vi "MB_PLC Comm Tester.vi"() -> ()   [LabVIEW 2018]
uses:
  Types/MB Ref Range_Cluster.ctl
  MB PLC Client.lvclass
  Data/MB Data Block.lvclass
  Types/MB Data Types_Enum.ctl
  Types/TCP Config_Cluster.ctl
  Types/PLC Config_Cluster.ctl
  Types/Serial Config_Cluster.ctl
  MB PLC Client.lvclass/MB PLC Client.ctl
  <vilib>/Plasmionique/MB Master/MB_ADU/MB_ADU.lvclass/MB_ADU.ctl
  Read MB session.vi
  <vilib>/Plasmionique/MB Master/MB_ADU/Read TX Data.vi
  <vilib>/Plasmionique/MB Master/MB_ADU/Read RX Data.vi
  <vilib>/Plasmionique/MB Master/MB_ADU/Read TX Timestamp.vi
  Read Poll List.vi
  c75dd57c-5bee-49d0-a77c-1ce558688484.vi
  28e4650d-529a-4e98-aa34-076f74409b59.vi
  46e13ee2-e094-4c5a-84fa-59b6ca3f2090.vi
  7f289292-5569-4f0d-9d85-fdf3f2f5d33f.vi
  734f5e53-c859-40ca-a5fa-c5cf108e6d6f.vi
  c81834c4-dabb-43f2-ab20-ca57d7a4baed.vi
  a754e2c8-79f3-43f7-b060-ecd024e2671e.vi
  Read PLC Config.vi
  0477ca1b-c906-4639-9e15-2d9a6e8c9738.vi
  7c55f3c8-79e0-44ec-bef0-26051c578f47.vi
  79f87e31-4c7f-45de-9eca-f5432d7d6e87.vi
  cd595503-730d-404a-9a2b-57208e76ed7d.vi
  b1a69734-ed15-4636-bb1c-7f177049bbcd.vi
  caadcf0a-5e3c-445f-9426-b9186ab7a80d.vi
  8821aff1-d05f-48ce-8825-efee275c2a12.vi
  Write Poll List.vi
  28e4650d-529a-4e98-aa34-076f74409b59.vi/fa59bfe1-0120-4885-ac93-9d9ea70f91fc.vi
  46e13ee2-e094-4c5a-84fa-59b6ca3f2090.vi/4d1e8f78-cfda-4438-959d-f24f6f91643b.vi
  7f289292-5569-4f0d-9d85-fdf3f2f5d33f.vi/b046c757-7f56-4393-a6ce-7771a5783ef5.vi
  734f5e53-c859-40ca-a5fa-c5cf108e6d6f.vi/f0ac0d71-d2d5-4ce4-9473-de91a0dd1fbe.vi
  c81834c4-dabb-43f2-ab20-ca57d7a4baed.vi/f658b24b-f49e-4e74-aef7-a7a595d7420c.vi
  a754e2c8-79f3-43f7-b060-ecd024e2671e.vi/da5e4fd7-561c-4cb8-8319-9a995167b5c8.vi
  0477ca1b-c906-4639-9e15-2d9a6e8c9738.vi/f491cc9f-02c6-4ff0-92db-d4c2192e9176.vi
  Read Data Block.vi
  7c55f3c8-79e0-44ec-bef0-26051c578f47.vi/6d4b17d2-94aa-44ea-9a19-d0a6b7bc1155.vi
  79f87e31-4c7f-45de-9eca-f5432d7d6e87.vi/0bbcd01c-01b7-4bc8-b012-ee89d531728c.vi
  cd595503-730d-404a-9a2b-57208e76ed7d.vi/d20b6ab7-2084-4e8d-b3bf-d366641d9b9f.vi
  b1a69734-ed15-4636-bb1c-7f177049bbcd.vi/f504e7b8-0e68-4180-b08b-6a52a05c8892.vi
  caadcf0a-5e3c-445f-9426-b9186ab7a80d.vi/238819c2-a843-4790-bae3-c60b5cb0f74c.vi
  8821aff1-d05f-48ce-8825-efee275c2a12.vi/d735e59b-17a8-402d-8d0a-4356da9fddb7.vi
  28e4650d-529a-4e98-aa34-076f74409b59.vi/fa59bfe1-0120-4885-ac93-9d9ea70f91fc.vi/6bf269be-e776-4970-9958-56c4dbea2623.vi
  46e13ee2-e094-4c5a-84fa-59b6ca3f2090.vi/4d1e8f78-cfda-4438-959d-f24f6f91643b.vi/79965a6c-bbeb-417c-a67a-cf8599a87570.vi
  7f289292-5569-4f0d-9d85-fdf3f2f5d33f.vi/b046c757-7f56-4393-a6ce-7771a5783ef5.vi/c7e8f3d7-7cb7-4e11-b1a0-06c415cc4c12.vi
  734f5e53-c859-40ca-a5fa-c5cf108e6d6f.vi/f0ac0d71-d2d5-4ce4-9473-de91a0dd1fbe.vi/b105db0b-c665-47de-b7cd-89c5a82b0a3a.vi
  c81834c4-dabb-43f2-ab20-ca57d7a4baed.vi/f658b24b-f49e-4e74-aef7-a7a595d7420c.vi/682b31c2-d550-4a42-88b0-f85749b69dfb.vi
  a754e2c8-79f3-43f7-b060-ecd024e2671e.vi/da5e4fd7-561c-4cb8-8319-9a995167b5c8.vi/d8f5afb1-d2bc-4e28-9ddd-dab29005bbc2.vi
  7c55f3c8-79e0-44ec-bef0-26051c578f47.vi/6d4b17d2-94aa-44ea-9a19-d0a6b7bc1155.vi/88869970-30da-475b-b9b2-9c3da2a1dedf.vi
  79f87e31-4c7f-45de-9eca-f5432d7d6e87.vi/0bbcd01c-01b7-4bc8-b012-ee89d531728c.vi/679bbca3-05f9-4675-a6af-c2baf730c5e7.vi
  cd595503-730d-404a-9a2b-57208e76ed7d.vi/d20b6ab7-2084-4e8d-b3bf-d366641d9b9f.vi/8995d4bf-6152-44d7-9e95-9528b4a066ce.vi
  b1a69734-ed15-4636-bb1c-7f177049bbcd.vi/f504e7b8-0e68-4180-b08b-6a52a05c8892.vi/fec356c3-a4ba-4058-8d4b-0e5c98c3ed52.vi
  caadcf0a-5e3c-445f-9426-b9186ab7a80d.vi/238819c2-a843-4790-bae3-c60b5cb0f74c.vi/1018f8a3-db30-48a7-bdd6-e7d4ad86f488.vi
  8821aff1-d05f-48ce-8825-efee275c2a12.vi/d735e59b-17a8-402d-8d0a-4356da9fddb7.vi/efbd7a58-b214-41d9-909a-8167e3be0071.vi
  <vilib>/Utility/error.llb/Error Cluster From Error Code.vi
  Write Coils_Cached.vi
  Write Holding Registers_Cached.vi
  <vilib>/Plasmionique/MB Master/MB_Master/MB_Master.lvclass
  <vilib>/Plasmionique/MB Master/MB_ADU/MB_ADU.lvclass
  MB PLC Client.lvlib
panel:
  out "Poll Count":u32
  out "Last Error Time":string
  in  "Tab Control 2":T1(tab)
  in  "Swap Words":bool
  in  "Reference Format":u16(ring)=5 items=["4 Digits"=4, "5 Digits"=5, "6 Digits"=6]
  in  "Open":bool
  in  "Close":bool
  in  "Type":enum16{"Serial", "TCP"}(ring) caption="Connection Type"
  in  "Tab Control":enum32{"Page 1", "Page 2"}(tab)
  in  "Retries":u8=1
  in  "Timeout (ms)":u32=300
  in  "Flow Control":u16(ring) items=["None", "XON/XOFF", "RTS/CTS", "XON/XOFF & RTS/CTS", "DTR/DSR", "XON/XOFF & DTR/DSR"]
  in  "Parity":u16(ring) items=["None", "Odd", "Even", "Mark", "Space"]
  in  "Stop Bits":u16(ring)=10 items=["1.0"=10, "1.5"=15, "2.0"=20]
  in  "Baud Rate (bps)":u32(ring)=19200 items=["9600"=9600, "19200"=19200, "38400"=38400, "57600"=57600, "115200"=115200, "460800"=460800, "921600"=921600]
  in  "Slave Address":u8=1
  in  "Mode":enum16{"RTU", "ASCII"}(ring)
  in  "COM Port":refnum<visa-resource-name>
  in  "TCP_Port":u16=502 caption="Port"
  in  "IP Address":string="localhost"
  in  "TCP_Timeout":i32=10000 caption="Timeout (ms)"
  in  "TCP_Slave ID":u8=255 caption="Slave ID" format="%.0x"
  in  "Poll Period (ms)":i32=1000
  in  "MaxPollGap":i32=1
  out "Message Log":T2(array[cluster]) {"dt" format="%d ms"; "Time" format="%<%H:%M:%S%1u>T"}
  out "Last Error Status":errorcluster
  out "Poll List":T3[](array[typedef])
  in  "New Value":dbl
  in  "Remove All":bool
  out "Register Type":string
  in  "Name":string
  in  "Data Type":T4(ring)
  in  "Starting Reference":u32 format="%05d"
  in  "Write Value":bool
  in  "Remove":bool
  in  "Add":bool
  in  "Watchlist":i32(listbox)
  out "Input Registers":u16[](array[numeric])
  out "Holding Registers":u16[](array[numeric]) format="%.0x"
  out "Discrete Inputs":bool[](array[boolean])
  out "Coils":bool[](array[boolean])
  out "Open?":bool caption="Connected"
  # "Communication Settngs"
  # "Communication Status"
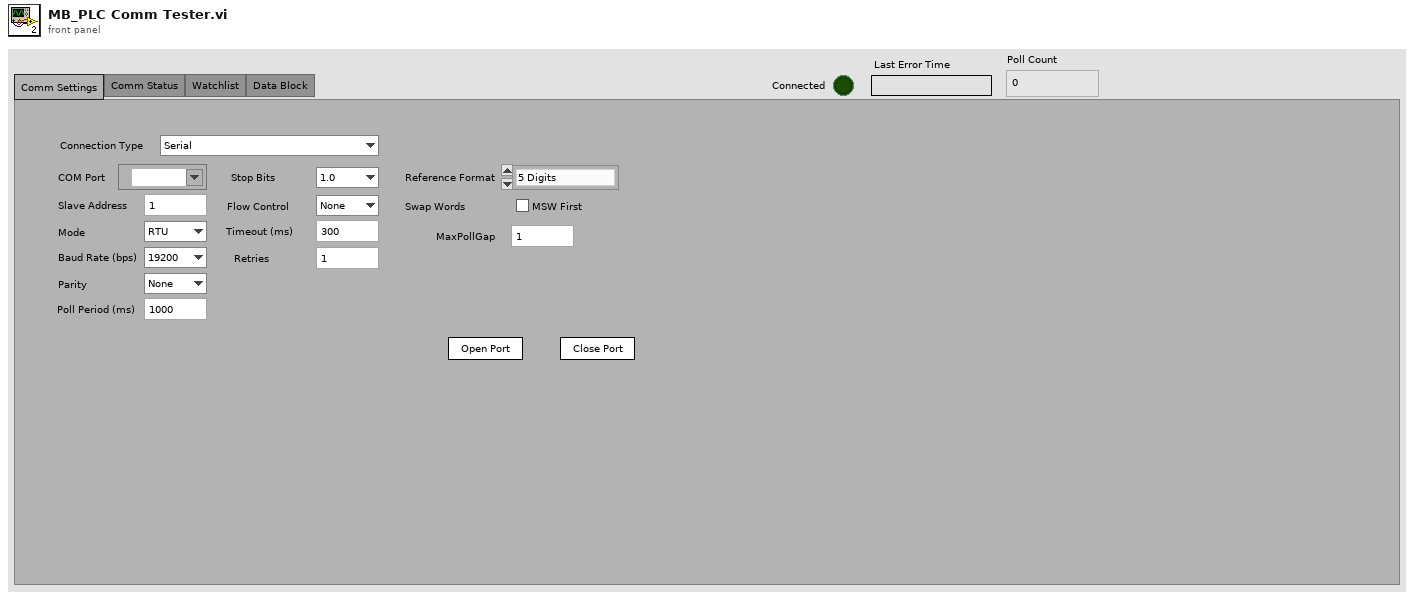
[diagram p1: front panel]
types:
  T1 = enum32{"Comm Settings", "Comm Status", "Watchlist", "Data Block"}
  T2 = cluster{"Time":timestamp, "TX":string, "RX":string, "dt":dbl}[]
  T3 = typedef "MB PLC Client.lvlib/MB Ref Range_Cluster.ctl" = cluster{"Start":u32, "Qty":u16}
  T4 = enum16{"Bool", "U16", "U32", "I16", "I32", "SGL", "DBL"}
  T5 = cluster{"Timestamp":timestamp, "TX":string, "RX":string, "dt":u32}
  T6 = typedef "MB PLC Client.lvlib/MB Data Types_Enum.ctl" = enum16{"Bool", "U16", "U32", "I16", "I32", "SGL", "DBL"}
  T7 = cluster{"Open":bool, "BinData":bool, "WatchList":cluster{"Name":string, "Reference":u32, "Data Type":T6, "Value":dbl}[], "Poll Count":u32}
  T8 = typedef "MB PLC Client.lvlib/Serial Config_Cluster.ctl" = cluster{"COM Port":string, "Slave ID":u8, "baud rate (bps)":u32, "Mode":enum16{"RTU", "ASCII"}, "Parity":u16, "Flow Control":u16, "Timeout":u32, "Retries":u8, "Stop Bits":u16}
  T9 = typedef "MB PLC Client.lvlib/PLC Config_Cluster.ctl" = cluster{"Use TCP":bool, "Reference Format":u16, "Swap Words":bool, "Poll List":T3[]}
  T10 = typedef "MB PLC Client.lvlib/TCP Config_Cluster.ctl" = cluster{"IP Address":string, "Port":u16, "Slave ID":i8, "Timeout":i32}
  T11 = cluster{"Name":string, "Reference":u32, "Data Type":T6, "Value":dbl}
  T12 = cluster{"Properties:TX Timestamp":timestamp, "string":string, "string":string, u32}
  T13 = cluster{"Name":string, "Reference":u32, "Data Type":T6, "Value":dbl}[]
  T14 = typedef "MB PLC Client.lvlib/Reference Types_Enum.ctl" = enum16{"Coil", "Discrete Input", "Input Register", "Holding Register", "Invalid"}
  T15 = cluster{"Timestamp":timestamp, "TX":string, "RX":string, "dt":u32}[]
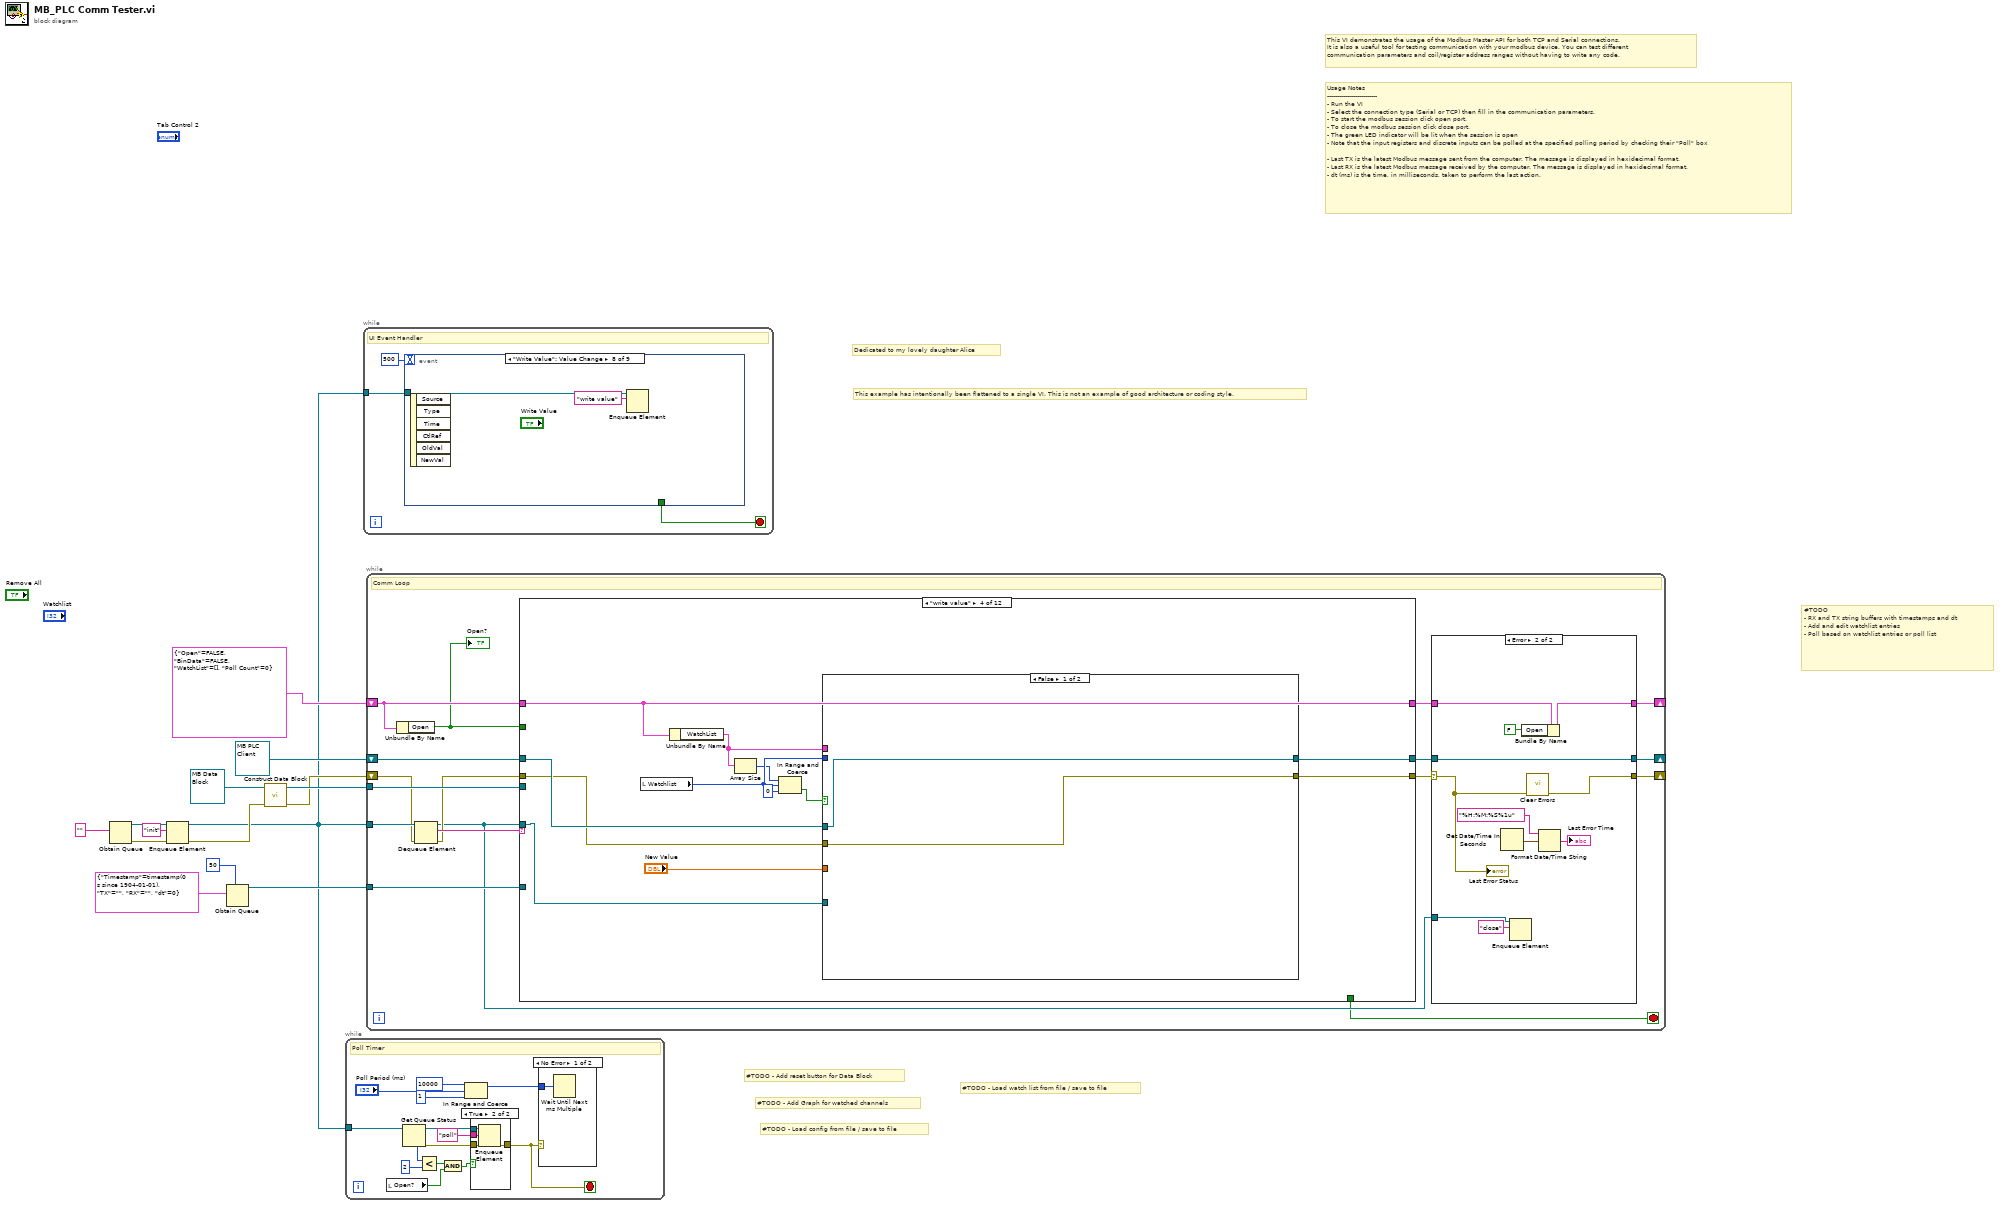
[diagram p0: block diagram]
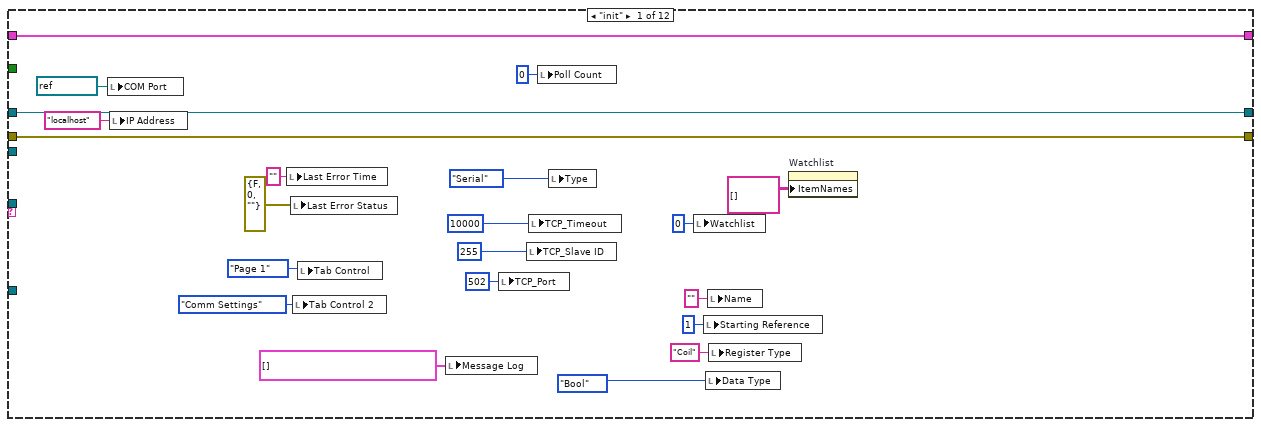
[diagram p5: hidden frame]
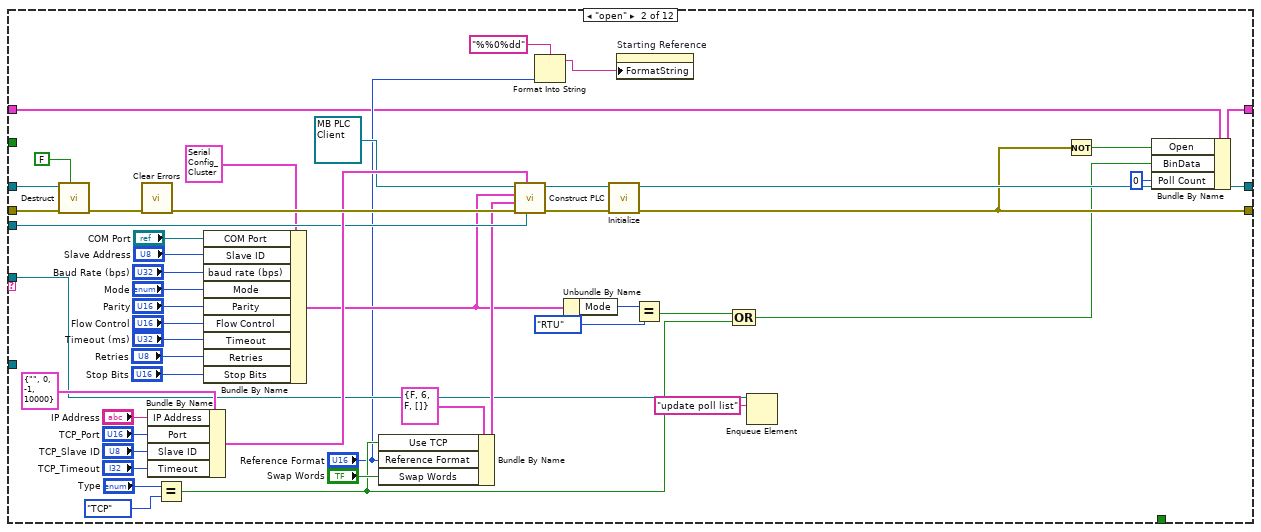
[diagram p6: hidden frame]
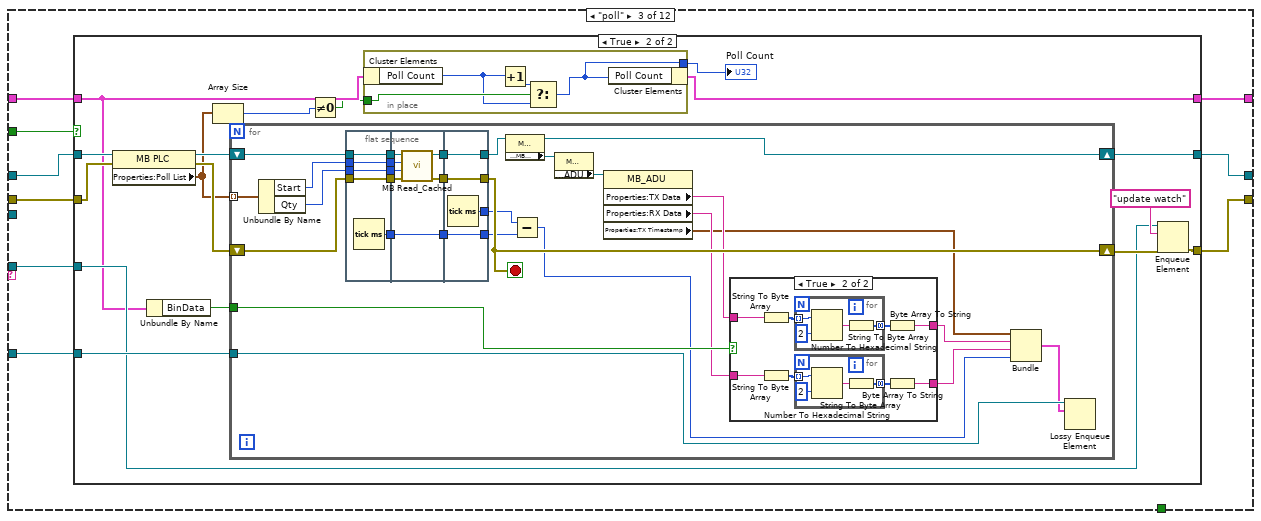
[diagram p7: hidden frame]
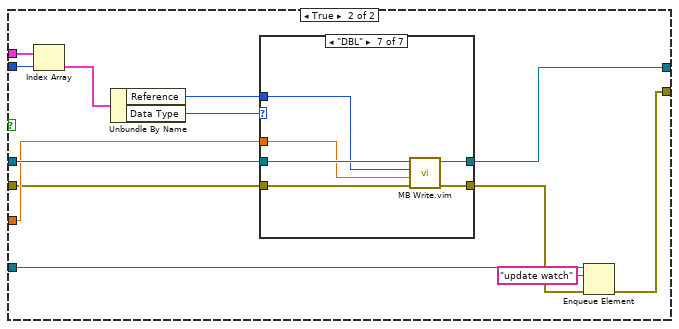
[diagram p10: hidden frame]
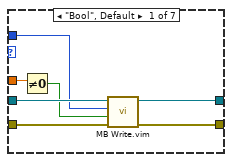
[diagram p11: hidden frame]
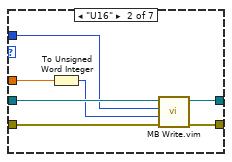
[diagram p12: hidden frame]
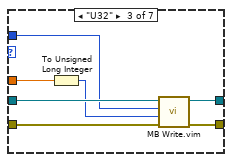
[diagram p13: hidden frame]
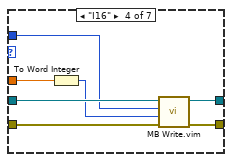
[diagram p14: hidden frame]
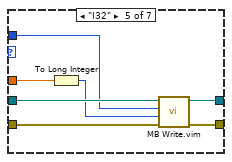
[diagram p15: hidden frame]
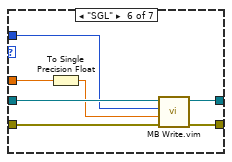
[diagram p16: hidden frame]
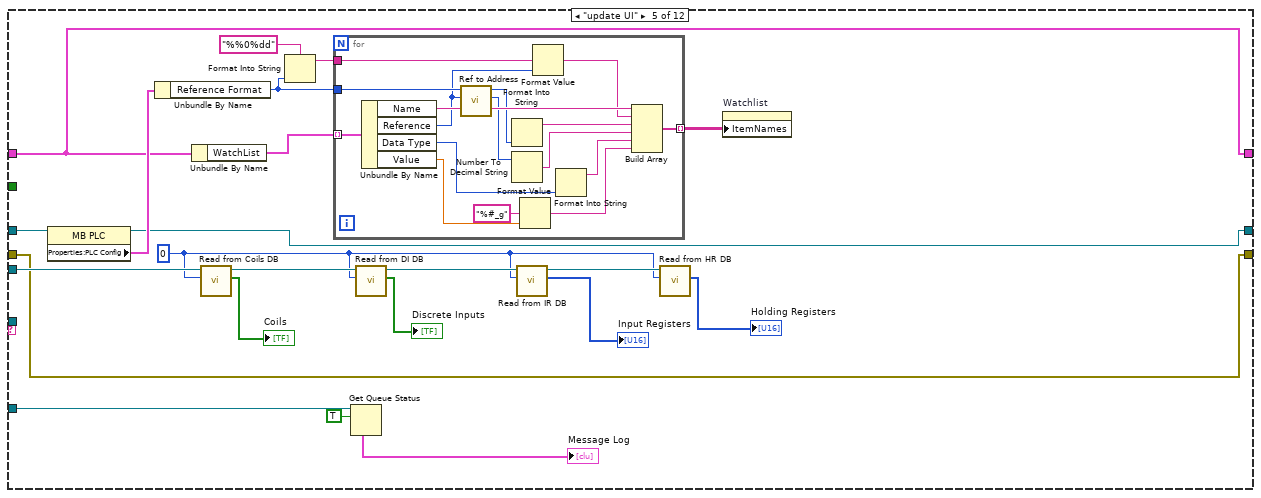
[diagram p17: hidden frame]
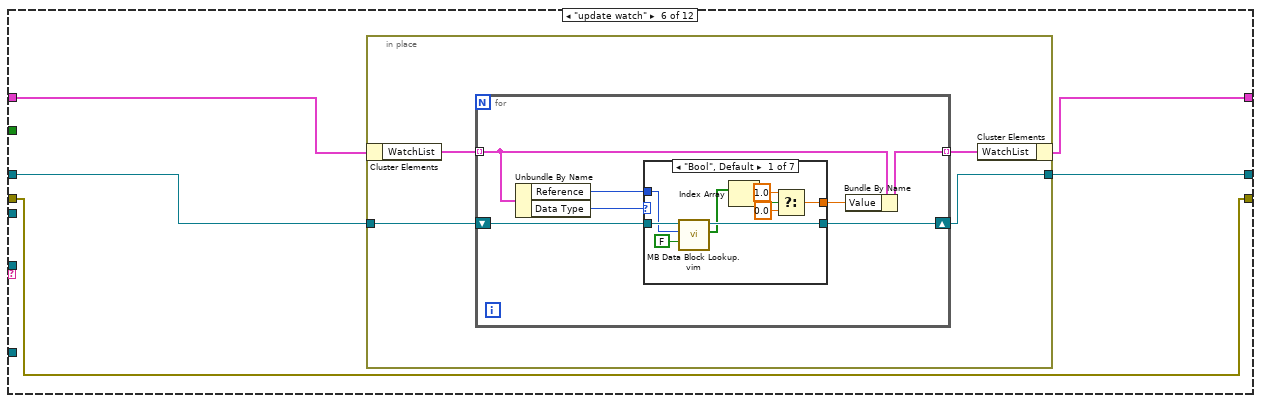
[diagram p18: hidden frame]
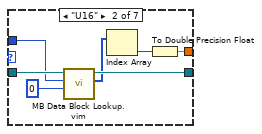
[diagram p19: hidden frame]
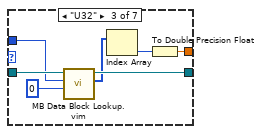
[diagram p20: hidden frame]
diagram:
  # "#TODO - Load watch list from file / save to file"
  # "#TODO - Load config from file / save to file"
  # "#TODO - Add Graph for watched channels"
  # "#TODO - Add reset button for Data Block"
  # "This example has intentionally been flattened to a single VI. This is not an example of good architecture or coding style."
  # "Dedicated to my lovely daughter Alice"
  # "#TODO\n- RX and TX string buffers with timestamps and dt\n- Add and edit watchlist entries\n- Poll based on watchlist entries or poll list"
  # "Usage Notes\n-------------------------\n- Run the VI\n- Select the connection type (Serial or TCP) then fill in the communication parameters.\n- To start the modbus session click open port.\n- To close the modbus session click close port.\n- The green LED indicator will be lit when the session is open\n- Note that the input registers and discrete inputs can be polled at the specified polling period by checking their \"Poll\" box\n\n- Last TX is the latest Modbus message sent from the computer. The message is displayed in hexidecimal format.\n- Last RX is the latest Modbus message received by the computer. The message is displayed in hexidecimal format. \n- dt (ms) is the time, in milliseconds, taken to perform the last action."
  # "This VI demonstrates the usage of the Modbus Master API for both TCP and Serial connections.\nIt is also a useful tool for testing communication with your modbus device. You can test different\ncommunication parameters and coil/register address ranges without having to write any code."
  n1 = Obtain Queue(element data type="") -> (queue out=w8:refnum<queue>, error out=w10:errorcluster)  [unwired: 4 in, 1 out]
  n2 = Enqueue Element(queue=w8, element="init", error in (no error)=w10) -> (queue out=w1:refnum<queue>, error out=w6:errorcluster)  [unwired: 1 in, 1 out]
  n3 = Obtain Queue(max queue size (-1, unlimited)=50, element data type=T5 {"Timestamp"=timestamp(0 s since 1904-01-01), "TX"="", "RX"="", "dt"=0}) -> (queue out=w2:refnum<queue>)  [unwired: 3 in, 2 out]
  n4 = call-dynamic "Construct Data Block.vi"("error in (no error)"=w6, "Modbus Data Store in"=refnum<class "MB Data Block.lvclass"> refnum ("MB Data Block (default)")) -> ("error out"=w5:errorcluster, "Modbus Data Store out"=w12:refnum<class "MB Data Block.lvclass">)  [unwired: 8 in]
  n5 = while {
    tunnel: w1 -> [w28]
    stop <- w19 stop-if-true
    # "Poll Timer"
    n6 = local read "Open?"() -> (w16:bool)
    n7 = Get Queue Status(queue=w28) -> (queue out=w20:refnum<queue>, error out=w21:errorcluster, # elements in queue=w27:i32)  [unwired: 2 in, 5 out]
    n8 = Less?(x=w27, y=2) -> (x < y?=w17:bool)
    n9 = And(x=w17, y=w16) -> (x .and. y?=w15:bool)
    n10 = In Range and Coerce(upper limit=10000, x="Poll Period (ms)", lower limit=1) -> (coerced(x)=w22:i32)  [unwired: 1 out]
    n11 = case shown="True" w15 {
      tunnel: w21 -> [w29 w33]
      tunnel: w20 -> [_ w32]
      tunnel: [w29 w31] -> w19
      tunnel: "poll" -> [_ w30]
      frame False {
      }
      frame True {
        n12 = Enqueue Element(queue=w32, element=w30, error in (no error)=w33) -> (error out=w31:errorcluster)  [unwired: 1 in, 2 out]
      }
    }
    n13 = case shown="No Error" w19 {
      tunnel: w22 -> [w34 _]
      frame No Error {
        n14 = Wait Until Next ms Multiple(millisecond multiple=w34) -> ()  [unwired: 1 out]
      }
      frame Error {
      }
    }
  }
  n15 = while {
    tunnel: w1 -> [w37]
    stop <- w36 stop-if-true
    # "UI Event Handler"
    n16 = event shown="[7] \"Write Value\": Value Change" {
      selector: _ -> [_ _ _ _ _ _ _ _ _]
      dyn-events: _ -> [_ _ _ _ _ _ _ _ _]
      timeout: 500 -> [_ _ _ _ _ _ _ _ _]
      tunnel: w37 -> [w38 w43 w46 w47 w49 w51 w53 w55 w57]
      tunnel: [_ _ _ _ _ _ _ _ TRUE] -> w36
      event Timeout {
        n17 = event-data() -> ()  [unwired: 1 in, 3 out]
        n18 = Enqueue Element(queue=w38, element="update UI") -> ()  [unwired: 2 in, 3 out]
      }
      event "Type": Value Change {
        # "Transparent (invisible) tab control contains comm parameter controls"
        # "Change connection type"
        n19 = event-data() -> ("NewVal"=w42:enum16{"Serial", "TCP"})  [unwired: 1 in, 5 out]
        n20 = Type Cast(type="Tab Control", x=w42) -> (*(type *) &x=w40:enum32{"Page 1", "Page 2"})
        n21 = local write "Tab Control"(w40) -> ()
        n22 = Enqueue Element(queue=w43, element="close") -> ()  [unwired: 2 in, 3 out]
      }
      event "Open": Value Change {
        # "Open modbus session"
        n23 = event-data() -> ()  [unwired: 1 in, 6 out]
        n24 = Enqueue Element(queue=w46, element="open") -> ()  [unwired: 2 in, 3 out]
      }
      event "Close": Value Change {
        # "Close modbus session"
        n25 = event-data() -> ()  [unwired: 1 in, 6 out]
        n26 = Enqueue Element(queue=w47, element="close") -> ()  [unwired: 2 in, 3 out]
      }
      event "Starting Reference", "Data Type": Value Change {
        n27 = event-data() -> ()  [unwired: 1 in, 6 out]
        n28 = Enqueue Element(queue=w49, element="validate watch") -> ()  [unwired: 2 in, 3 out]
      }
      event "Add": Value Change {
        n29 = event-data() -> ()  [unwired: 1 in, 6 out]
        n30 = Enqueue Element(queue=w51, element="add watch") -> ()  [unwired: 2 in, 3 out]
      }
      event "Remove": Value Change {
        n31 = event-data() -> ()  [unwired: 1 in, 6 out]
        n32 = Enqueue Element(queue=w53, element="remove watch") -> ()  [unwired: 2 in, 3 out]
      }
      event "Write Value": Value Change {
        n33 = event-data() -> ()  [unwired: 1 in, 6 out]
        n34 = Enqueue Element(queue=w55, element="write value") -> ()  [unwired: 2 in, 3 out]
      }
      event Panel Close? {
        n35 = event-data() -> ()  [unwired: 1 in, 4 out]
        n36 = Enqueue Element(queue=w57, element="shutdown") -> ()  [unwired: 2 in, 3 out]
        n37 = event-data("Discard?"=TRUE) -> ()  [unwired: 1 in, 1 out]
      }
    }
  }
  n38 = while {
    shift-right: [w62] -> _
    shift-left: refnum<class "MB PLC Client.lvclass"> refnum ("PLC in") -> [w77]
    tunnel: w12 -> [w76]
    shift-right: [w65] -> _
    shift-left: w5 -> [w67]
    shift-right: [w63] -> _
    shift-left: T7 {"Open"=FALSE, "BinData"=FALSE, "WatchList"=[], "Poll Count"=0} -> [w74]
    tunnel: w1 -> [w75]
    tunnel: w2 -> [w72]
    stop <- w61 stop-if-true
    # "Comm Loop"
    n39 = Unbundle By Name(w74) -> ("Open"=w73:bool)
    "Open?" <- w73
    n40 = Dequeue Element(queue=w75, error in (no error)=w67) -> (queue out=w64:refnum<queue>, element=w71:string, error out=w66:errorcluster)  [unwired: 1 in, 1 out]
    n41 = case shown="\"write value\"" w71 {
      tunnel: w77 -> [w101 w149 w167 w267 w339 w373 w440 w471 w488 w497 w508 w518]
      tunnel: w76 -> [_ w146 _ _ w349 _ _ _ _ _ _ _]
      tunnel: [w101 w140 w165 w265 w332 w371 w439 w471 w480 w493 w507 refnum<class "MB PLC Client.lvclass"> refnum ("PLC out")] -> w68
      tunnel: [w100 w127 w161 w261 w333 w370 w444 w467 w479 w492 w506 w514] -> w70
      tunnel: w74 -> [w102 w114 w164 w263 w331 w372 w450 w475 w489 w494 w511 w519]
      tunnel: [w102 w128 w163 w263 w331 w369 w445 w474 w489 w494 w509 w519] -> w69
      tunnel: w66 -> [w100 w126 w166 w264 w333 w370 w444 w467 w479 w496 w505 w517]
      tunnel: w64 -> [_ w118 w160 w262 _ _ w435 w470 _ _ _ w513]
      tunnel: w73 -> [_ _ w168 _ _ _ _ _ _ _ _ _]
      tunnel: w72 -> [_ _ w162 _ w352 _ _ _ _ _ _ w512]
      tunnel: [_ _ _ _ _ _ _ _ _ _ _ TRUE] -> w61
      frame "init" {
        n42 = local write "COM Port"(refnum<visa-resource-name> refnum ("COM Port")) -> ()
        n43 = local write "IP Address"("localhost" ("IP Address")) -> ()
        n44 = local write "Last Error Time"("" ("Last Error Time")) -> ()
        n45 = local write "Last Error Status"(errorcluster {"status"=FALSE, "code"=0, "source"=""} ("Last Error Status")) -> ()
        n46 = local write "Tab Control 2"(enum32{"Comm Settings", "Comm Status"}."Comm Settings" ("Tab Control 2")) -> ()
        n47 = local write "Tab Control"(enum32{"Page 1", "Page 2"}."Page 1" ("Tab Control")) -> ()
        n48 = local write "Message Log"(T2 [] ("Message Log")) -> ()
        n49 = local write "TCP_Port"(u16 502 ("TCP_Port")) -> ()
        n50 = local write "TCP_Slave ID"(u8 255 ("TCP_Slave ID")) -> ()
        n51 = local write "TCP_Timeout"(10000 ("TCP_Timeout")) -> ()
        n52 = local write "Poll Count"(u32 0 ("Poll Count")) -> ()
        n53 = local write "Type"(enum16{"Serial", "TCP"}."Serial" ("Type")) -> ()
        n54 = local write "Watchlist"(0 ("Watchlist")) -> ()
        n55 = local write "Starting Reference"(u32 1 ("Starting Reference")) -> ()
        n56 = local write "Data Type"(MB_Data_Types_Enum."Bool" ("Data Type")) -> ()
        n57 = local write "Name"("" ("Name")) -> ()
        n58 = local write "Register Type"("Coil" ("Register Type")) -> ()
        n59 = property on="Watchlist" class="MCListbox (strict)"("ItemNames"=string[][] [] ("Item Names")) -> ()  [unwired: 2 in, 2 out]
      }
      frame "open" {
        n60 = call-dynamic "Destruct.vi"("Destroy Data Block? (t)"=FALSE, "error in (no error)"=w126, "PLC in"=w149) -> ("error out"=w148:errorcluster)  [unwired: 8 in]
        n61 = call <vilib>:"Clear Errors.vi"("error in (no error)"=w148) -> ("error out"=w157:errorcluster)  [unwired: 5 in, 1 out]
        n62 = Bundle By Name(cluster=T10 {"IP Address"="", "Port"=0, "Slave ID"=-1, "Timeout"=10000} ("TCP Config"), "IP Address"="IP Address", "Port"="TCP_Port", "Slave ID"="TCP_Slave ID", "Timeout"="TCP_Timeout") -> (w151:T10)
        n63 = Equal?(x="Type", y=enum16{"Serial", "TCP"}."TCP") -> (x = y?=w121:bool)
        n64 = Bundle By Name(cluster=T8 {"COM Port"="COM1", "Slave ID"=1, "baud rate (bps)"=460800, "Mode"=enum."RTU", "Parity"=0, "Flow Control"=0, "Timeout"=200, "Retries"=1, "Stop Bits"=10} ("Serial Config"), "COM Port"="COM Port", "Slave ID"="Slave Address", "baud rate (bps)"="Baud Rate (bps)", "Mode"="Mode", "Parity"="Parity", "Flow Control"="Flow Control", "Timeout"="Timeout (ms)", "Retries"="Retries", "Stop Bits"="Stop Bits") -> (w125:T8)
        n65 = Bundle By Name(cluster=T9 {"Use TCP"=FALSE, "Reference Format"=6, "Swap Words"=FALSE, "Poll List"=[]} ("PLC Config"), "Use TCP"=w121, "Reference Format"="Reference Format", "Swap Words"="Swap Words") -> (w142:T9)
        n66 = call-dynamic "Construct PLC.vi"("MB Data Block (default)"=w146, "TCP Config"=w151, "error in (no error)"=w157, "PLC Config"=w142, "Serial Config"=w125, "PLC in"=refnum<class "MB PLC Client.lvclass"> refnum) -> ("error out"=w143:errorcluster, "PLC out"=w144:refnum<class "MB PLC Client.lvclass">)  [unwired: 4 in]
        n67 = Format Into String(format string="%%0%dd", "Reference Format") -> (resulting string=w115:string)  [unwired: 2 in, 1 out]
        n68 = Unbundle By Name(w125) -> ("Mode"=w124:enum16{"RTU", "ASCII"})
        n69 = call-dynamic "Initialize.vi"("error in (no error)"=w143, "PLC in"=w144) -> ("error out"=w127:errorcluster, "PLC out"=w140:refnum<class "MB PLC Client.lvclass">)  [unwired: 8 in]
        n70 = property on="Starting Reference" class="DigNum (strict)"("FormatString"=w115) -> ()  [unwired: 2 in, 2 out]
        n71 = Equal?(x=w124, y=enum16{"RTU", "ASCII"}."RTU") -> (x = y?=w122:bool)
        n72 = Compound Arithmetic op=OR(w122, w121) -> (w120:bool)
        n73 = Enqueue Element(queue=w118, element="update poll list") -> ()  [unwired: 2 in, 3 out]
        n74 = Not(x=w127) -> (.not. x?=w129:bool)
        n75 = Bundle By Name(cluster=w114, "Open"=w129, "BinData"=w120, "Poll Count"=u32 0) -> (w128:T7)
      }
      frame "poll" {
        n76 = case shown="True" w168 {
          tunnel: w167 -> [w171 w187]
          tunnel: [w171 w188] -> w165
          tunnel: [w170 w179] -> w161
          tunnel: w166 -> [w170 w185]
          tunnel: w164 -> [w169 w177]
          tunnel: [w169 w176] -> w163
          tunnel: w162 -> [_ w182]
          tunnel: w160 -> [_ w178]
          frame False {
          }
          frame True {
            n77 = property class="MB PLC"(reference=w187, error in=w185) -> (reference out=w186:refnum<class "MB PLC Client.lvclass">, error out=w184:errorcluster, "Properties:Poll List"=w174:T3[])
            n78 = Unbundle By Name(w177) -> ("BinData"=w183:bool)
            n79 = Array Size(array=w174) -> (size(s)=w173:i32)
            n80 = for {
              shift-right: [w202] -> w188
              shift-left: w186 -> [w221]
              tunnel: w174 -> [w220] mode=indexing
              shift-right: [w216] -> w180
              shift-left: w184 -> [w217]
              tunnel: w183 -> [w200]
              tunnel: w182 -> [w194]
              stop <- w216 stop-if-true
              n81 = Unbundle By Name(w220) -> ("Start"=w219:u32, "Qty"=w218:u16)
              n82 = flat-sequence {
                tunnel: w217 -> [w241]
                tunnel: w218 -> [w242]
                tunnel: w219 -> [w243]
                tunnel: w221 -> [w244]
                tunnel: [w244] -> w215
                tunnel: [w243] -> w214
                tunnel: [w242] -> w213
                tunnel: [w241] -> w212
                tunnel: [w240] -> w208
                tunnel: w215 -> [w251]
                tunnel: w214 -> [w249]
                tunnel: w213 -> [w248]
                tunnel: w212 -> [w247]
                tunnel: [w250] -> w211
                tunnel: [w246] -> w210
                tunnel: [w245] -> w209
                tunnel: w208 -> [w245]
                tunnel: [w254] -> w216
                tunnel: [w255] -> w207
                tunnel: w211 -> [w255]
                tunnel: w210 -> [w254]
                tunnel: [w253] -> w203
                tunnel: w209 -> [w253]
                tunnel: [w252] -> w204
                frame #0 {
                  n83 = Tick Count (ms)() -> (millisecond timer value=w240:u32)
                }
                frame #1 {
                  n84 = call "MB Read_Cached.vi"("error in (no error)"=w247, "Quantity(1)"=w248, "Modbus Reference"=w249, "MB PLC in"=w251) -> ("error out"=w246:errorcluster, "MB PLC out"=w250:refnum<class "MB PLC Client.lvclass">)  [unwired: 6 in]
                }
                frame #2 {
                  n85 = Tick Count (ms)() -> (millisecond timer value=w252:u32)
                }
              }
              n86 = property class="MB PLC"(reference=w207) -> (reference out=w202:refnum<class "MB PLC Client.lvclass">, "Properties:MB session"=w206:refnum<class "MB_Master.lvclass">)  [unwired: 1 in, 1 out]
              n87 = Subtract(x=w204, y=w203) -> (x-y=w195:u32)
              n88 = property class="MB_Master"(reference=w206) -> ("Properties:ADU"=w205:refnum<class "MB_ADU.lvclass">)  [unwired: 1 in, 2 out]
              n89 = property class="MB_ADU"(reference=w205) -> ("Properties:TX Data"=w201:string, "Properties:RX Data"=w199:string, "Properties:TX Timestamp"=w197:timestamp)  [unwired: 1 in, 2 out]
              n90 = case shown="True" w200 {
                tunnel: w201 -> [w223 w227]
                tunnel: w199 -> [w222 w226]
                tunnel: [w223 w225] -> w198
                tunnel: [w222 w224] -> w196
                frame False {
                }
                frame True {
                  n91 = String To Byte Array(string=w227) -> (unsigned byte array=w230:u8[])
                  n92 = String To Byte Array(string=w226) -> (unsigned byte array=w229:u8[])
                  n93 = for {
                    tunnel: w230 -> [w239] mode=indexing
                    tunnel: [w237] -> w231 mode=concatenating
                    n94 = Number To Hexadecimal String(1:i16 2 ("width (-)"), 2:w239) -> (0:w236:string)
                    n95 = String To Byte Array(string=w236) -> (unsigned byte array=w237:u8[])
                  }
                  n96 = for {
                    tunnel: w229 -> [w235] mode=indexing
                    tunnel: [w233] -> w228 mode=concatenating
                    n97 = Number To Hexadecimal String(1:i16 2 ("width (-)"), 2:w235) -> (0:w232:string)
                    n98 = String To Byte Array(string=w232) -> (unsigned byte array=w233:u8[])
                  }
                  n99 = Byte Array To String(unsigned byte array=w231) -> (string=w225:string)
                  n100 = Byte Array To String(unsigned byte array=w228) -> (string=w224:string)
                }
              }
              n101 = Bundle("Properties:TX Timestamp"=w197, "string"=w198, "string"=w196, w195) -> (w193:T12)  [unwired: 1 in]
              n102 = Lossy Enqueue Element(queue=w194, element=w193) -> ()  [unwired: 1 in, 4 out]
            }
            n103 = Not Equal To 0?(x=w173) -> (x != 0?=w172:bool)
            n104 = in-place {
              in-place-border: [w189] -> w175
              in-place-border: w172 -> [w192]
              n105 = in-place-cluster #1(w177) -> ("Poll Count"=w191:u32)
              n106 = Increment(x=w191) -> (x+1=w190:u32)
              n107 = Select(t=w190, s=w192, f=w191) -> (s? t:f=w189:u32)
              n108 = in-place-cluster #1("Poll Count"=w189) -> (w176:T7)
            }
            "Poll Count" <- w175
            n109 = Enqueue Element(queue=w178, element="update watch", error in (no error)=w180) -> (error out=w179:errorcluster)  [unwired: 1 in, 2 out]
          }
        }
      }
      frame "write value" {
        n110 = local read "Watchlist"() -> (w259:i32)
        n111 = Unbundle By Name(w263) -> ("WatchList"=w260:T13)
        n112 = Array Size(array=w260) -> (size(s)=w257:i32)
        n113 = In Range and Coerce(upper limit=w257, x=w259, lower limit=0) -> (In Range?=w256:bool)  [unwired: 1 out]
        n114 = case shown="False" w256 {
          tunnel: w260 -> [_ w282]
          tunnel: w259 -> [_ w281]
          tunnel: w267 -> [w269 w279]
          tunnel: "New Value" -> [_ w276]
          tunnel: [w269 w275] -> w265
          tunnel: w264 -> [w268 w274]
          tunnel: w262 -> [_ w272]
          tunnel: [w268 w270] -> w261
          frame False {
          }
          frame True {
            n115 = Index Array(array=w282, index=w281) -> (element=w280:T11)
            n116 = Unbundle By Name(w280) -> ("Reference"=w277:u32, "Data Type"=w278:T6)
            n117 = case shown="\"DBL\"" w278 {
              tunnel: w279 -> [w288 w296 w303 w310 w317 w324 w330]
              tunnel: w277 -> [w287 w292 w299 w306 w313 w320 w326]
              tunnel: w276 -> [w289 w291 w298 w305 w312 w319 w325]
              tunnel: [w285 w294 w301 w308 w315 w322 w328] -> w275
              tunnel: w274 -> [w284 w295 w302 w309 w316 w323 w329]
              tunnel: [w283 w293 w300 w307 w314 w321 w327] -> w271
              frame "Bool", Default {
                n118 = Not Equal To 0?(x=w289) -> (x != 0?=w286:bool)
                n119 = call "MB Write.vim"("error in (no error)"=w284, "Value"=w286, "Modbus Reference"=w287, "MB PLC in"=w288) -> ("error out"=w283:errorcluster, "MB PLC out"=w285:refnum<class "MB PLC Client.lvclass">)  [unwired: 6 in]
              }
              frame "U16" {
                n120 = To Unsigned Word Integer(number=w291) -> (unsigned 16bit integer=w290:u16)
                n121 = call "MB Write.vim"("error in (no error)"=w295, "Value"=w290, "Modbus Reference"=w292, "MB PLC in"=w296) -> ("error out"=w293:errorcluster, "MB PLC out"=w294:refnum<class "MB PLC Client.lvclass">)  [unwired: 6 in]
              }
              frame "U32" {
                n122 = To Unsigned Long Integer(number=w298) -> (unsigned 32bit integer=w297:u32)
                n123 = call "MB Write.vim"("error in (no error)"=w302, "Value"=w297, "Modbus Reference"=w299, "MB PLC in"=w303) -> ("error out"=w300:errorcluster, "MB PLC out"=w301:refnum<class "MB PLC Client.lvclass">)  [unwired: 6 in]
              }
              frame "I16" {
                n124 = To Word Integer(number=w305) -> (16bit integer=w304:i16)
                n125 = call "MB Write.vim"("error in (no error)"=w309, "Value"=w304, "Modbus Reference"=w306, "MB PLC in"=w310) -> ("error out"=w307:errorcluster, "MB PLC out"=w308:refnum<class "MB PLC Client.lvclass">)  [unwired: 6 in]
              }
              frame "I32" {
                n126 = To Long Integer(number=w312) -> (32bit integer=w311:i32)
                n127 = call "MB Write.vim"("error in (no error)"=w316, "Value"=w311, "Modbus Reference"=w313, "MB PLC in"=w317) -> ("error out"=w314:errorcluster, "MB PLC out"=w315:refnum<class "MB PLC Client.lvclass">)  [unwired: 6 in]
              }
              frame "SGL" {
                n128 = To Single Precision Float(number=w319) -> (single precision float=w318:sgl)
                n129 = call "MB Write.vim"("error in (no error)"=w323, "Value"=w318, "Modbus Reference"=w320, "MB PLC in"=w324) -> ("error out"=w321:errorcluster, "MB PLC out"=w322:refnum<class "MB PLC Client.lvclass">)  [unwired: 6 in]
              }
              frame "DBL" {
                n130 = call "MB Write.vim"("error in (no error)"=w329, "Value"=w325, "Modbus Reference"=w326, "MB PLC in"=w330) -> ("error out"=w327:errorcluster, "MB PLC out"=w328:refnum<class "MB PLC Client.lvclass">)  [unwired: 6 in]
              }
            }
            n131 = Enqueue Element(queue=w272, element="update watch", error in (no error)=w271) -> (error out=w270:errorcluster)  [unwired: 1 in, 2 out]
          }
        }
      }
      frame "update UI" {
        w341 = u16 0 ("Modbus Address")
        n132 = property class="MB PLC"(reference=w339) -> (reference out=w332:refnum<class "MB PLC Client.lvclass">, "Properties:PLC Config"=w338:T9)  [unwired: 1 in, 1 out]
        n133 = Unbundle By Name(w338) -> ("Reference Format"=w337:u16)
        n134 = Unbundle By Name(w331) -> ("WatchList"=w340:T13)
        n135 = call-dynamic "Read from Coils DB.vi"("Modbus Address"=w341, "MB Data Block in"=w349) -> ("Data out"=→"Coils":bool[], "MB Data Block out"=w348:refnum<class "MB Data Block.lvclass">)  [unwired: 7 in, 1 out]
        n136 = Format Into String(format string="%%0%dd", w337) -> (resulting string=w335:string)  [unwired: 2 in, 1 out]
        n137 = for {
          tunnel: w340 -> [w368] mode=indexing
          tunnel: w337 -> [w354]
          tunnel: [w364] -> w334 mode=indexing
          tunnel: w335 -> [w360]
          n138 = Unbundle By Name(w368) -> ("Name"=w367:string, "Reference"=w353:u32, "Data Type"=w363:T6, "Value"=w366:dbl)
          n139 = call "Ref to Address.vi"("Reference"=w353, "Reference Format"=w354) -> ("Address"=w357:u16, "Reference Type"=w361:T14)  [unwired: 8 in]
          n140 = Format Into String(w361) -> (resulting string=w358:string)  [unwired: 3 in, 1 out]
          n141 = Number To Decimal String(number=w357) -> (decimal integer string=w356:string)  [unwired: 1 in]
          n142 = Format Value(format string="%#_g", value (0)=w366) -> (output string=w365:string)  [unwired: 1 in]
          n143 = Format Value(format string=w360, value (0)=w353) -> (output string=w359:string)  [unwired: 1 in]
          n144 = Format Into String(w363) -> (resulting string=w362:string)  [unwired: 3 in, 1 out]
          n145 = Build Array(w367, w359, w358, w356, w362, w365) -> (w364:string[])
        }
        n146 = Get Queue Status(queue=w352, return elements? (F)=TRUE) -> (elements=→"Message Log":T15)  [unwired: 1 in, 7 out]
        n147 = call-dynamic "Read from DI DB.vi"("Modbus Address"=w341, "MB Data Block in"=w348) -> ("Data out"=→"Discrete Inputs":bool[], "MB Data Block out"=w345:refnum<class "MB Data Block.lvclass">)  [unwired: 7 in, 1 out]
        n148 = call-dynamic "Read from IR DB.vi"("Modbus Address"=w341, "MB Data Block in"=w345) -> ("Data out"=→"Input Registers":u16[], "MB Data Block out"=w344:refnum<class "MB Data Block.lvclass">)  [unwired: 7 in, 1 out]
        n149 = call-dynamic "Read from HR DB.vi"("Modbus Address"=w341, "MB Data Block in"=w344) -> ("Data out"=→"Holding Registers":u16[])  [unwired: 7 in, 2 out]
        n150 = property on="Watchlist" class="MCListbox (strict)"("ItemNames"=w334) -> ()  [unwired: 2 in, 2 out]
      }
      frame "update watch" {
        n151 = in-place {
          in-place-border: w373 -> [w377]
          in-place-border: [w374] -> w371
          n152 = in-place-cluster #2(w372) -> ("WatchList"=w376:T13)
          n153 = for {
            tunnel: w376 -> [w383] mode=indexing
            shift-right: [w379] -> w374
            shift-left: w377 -> [w384]
            tunnel: [w380] -> w375 mode=indexing
            n154 = Unbundle By Name(w383) -> ("Reference"=w381:u32, "Data Type"=w382:T6)
            n155 = case shown="\"Bool\", Default" w382 {
              tunnel: w384 -> [w393 w400 w407 w414 w421 w428 w434]
              tunnel: w381 -> [w391 w399 w406 w413 w420 w427 w433]
              tunnel: [w392 w397 w404 w411 w418 w425 w431] -> w379
              tunnel: [w387 w394 w401 w408 w415 w422 w429] -> w378
              frame "Bool", Default {
                n156 = call "MB Data Block Lookup.vim"("Type"=FALSE, "Modbus Reference"=w391, "MB PLC in"=w393) -> ("Data out"=w389:bool[], "MB PLC out"=w392:refnum<class "MB PLC Client.lvclass">)  [unwired: 6 in, 1 out]
                n157 = Index Array(array=w389) -> (element=w388:bool)  [unwired: 1 in]
                n158 = Select(t=1.0, s=w388, f=0.0) -> (s? t:f=w387:dbl)
              }
              frame "U16" {
                n159 = call "MB Data Block Lookup.vim"("Type"=u16 0, "Modbus Reference"=w399, "MB PLC in"=w400) -> ("Data out"=w396:u16[], "MB PLC out"=w397:refnum<class "MB PLC Client.lvclass">)  [unwired: 6 in, 1 out]
                n160 = Index Array(array=w396) -> (element=w395:u16)  [unwired: 1 in]
                n161 = To Double Precision Float(number=w395) -> (double precision float=w394:dbl)
              }
              frame "U32" {
                n162 = call "MB Data Block Lookup.vim"("Type"=u32 0, "Modbus Reference"=w406, "MB PLC in"=w407) -> ("Data out"=w403:u32[], "MB PLC out"=w404:refnum<class "MB PLC Client.lvclass">)  [unwired: 6 in, 1 out]
                n163 = Index Array(array=w403) -> (element=w402:u32)  [unwired: 1 in]
                n164 = To Double Precision Float(number=w402) -> (double precision float=w401:dbl)
              }
              frame "I16" {
                n165 = call "MB Data Block Lookup.vim"("Type"=i16 0, "Modbus Reference"=w413, "MB PLC in"=w414) -> ("Data out"=w410:i16[], "MB PLC out"=w411:refnum<class "MB PLC Client.lvclass">)  [unwired: 6 in, 1 out]
                n166 = Index Array(array=w410) -> (element=w409:i16)  [unwired: 1 in]
                n167 = To Double Precision Float(number=w409) -> (double precision float=w408:dbl)
              }
              frame "I32" {
                n168 = call "MB Data Block Lookup.vim"("Type"=0, "Modbus Reference"=w420, "MB PLC in"=w421) -> ("Data out"=w417:i32[], "MB PLC out"=w418:refnum<class "MB PLC Client.lvclass">)  [unwired: 6 in, 1 out]
                n169 = Index Array(array=w417) -> (element=w416:i32)  [unwired: 1 in]
                n170 = To Double Precision Float(number=w416) -> (double precision float=w415:dbl)
              }
              frame "SGL" {
                n171 = call "MB Data Block Lookup.vim"("Type"=sgl 0.0, "Modbus Reference"=w427, "MB PLC in"=w428) -> ("Data out"=w424:sgl[], "MB PLC out"=w425:refnum<class "MB PLC Client.lvclass">)  [unwired: 6 in, 1 out]
                n172 = Index Array(array=w424) -> (element=w423:sgl)  [unwired: 1 in]
                n173 = To Double Precision Float(number=w423) -> (double precision float=w422:dbl)
              }
              frame "DBL" {
                n174 = call "MB Data Block Lookup.vim"("Type"=0.0, "Modbus Reference"=w433, "MB PLC in"=w434) -> ("Data out"=w430:dbl[], "MB PLC out"=w431:refnum<class "MB PLC Client.lvclass">)  [unwired: 6 in, 1 out]
                n175 = Index Array(array=w430) -> (element=w429:dbl)  [unwired: 1 in]
              }
            }
            n176 = Bundle By Name(cluster=w383, "Value"=w378) -> (w380:T11)
          }
          n177 = in-place-cluster #2("WatchList"=w375) -> (w369:T7)
        }
      }
      frame "add watch" {
        n178 = property class="MB PLC"(reference=w440) -> (reference out=w439:refnum<class "MB PLC Client.lvclass">, "Properties:PLC Config"=w438:T9)  [unwired: 1 in, 1 out]
        n179 = Unbundle By Name(w438) -> ("Reference Format"=w437:u16)
        n180 = local read "Watchlist"() -> (w442:i32)
        n181 = call "Ref to Address.vi"("Reference"="Starting Reference", "Reference Format"=w437) -> ("Reference Type"=w436:T14)  [unwired: 8 in, 1 out]
        n182 = Bundle By Name(cluster=T11 {"Name"="", "Reference"=0, "Data Type"=enum."Bool", "Value"=0.0} ("new element/subarray"), "Name"="Name", "Reference"="Starting Reference", "Data Type"="Data Type", "Value"=nan) -> (w446:T11)
        n183 = case shown="\"Discrete Input\", Default" w436 {
          tunnel: w450 -> [w451 w459]
          tunnel: w446 -> [_ w458]
          tunnel: [w451 w457] -> w445
          tunnel: w442 -> [_ w456]
          tunnel: w435 -> [_ w452]
          frame "Invalid" {
          }
          frame "Discrete Input", Default {
            n184 = in-place {
              in-place-border: w458 -> [w465]
              in-place-border: w456 -> [w464]
              n185 = in-place-cluster #3(w459) -> ("WatchList"=w462:T13)
              n186 = Array Size(array=w462) -> (size(s)=w461:i32)
              n187 = In Range and Coerce(upper limit=w461, x=w464, lower limit=0) -> (coerced(x)=w460:i32)  [unwired: 1 out]
              n188 = Insert Into Array(array=w462, index=w460, new element=w465) -> (w466:T13)
              n189 = in-place-cluster #3("WatchList"=w466) -> (w457:T7)
            }
            n190 = Enqueue Element(queue=w452, element="update poll list") -> (queue out=w455:refnum<queue>)  [unwired: 2 in, 2 out]
            n191 = Enqueue Element(queue=w455, element="update UI") -> ()  [unwired: 2 in, 3 out]
          }
        }
      }
      frame "remove watch" {
        n192 = local read "Watchlist"() -> (w473:i32)
        n193 = in-place {
          in-place-border: w473 -> [w476]
          n194 = in-place-cluster #4(w475) -> ("WatchList"=w478:T13)
          n195 = Delete From Array(array=w478, index=w476) -> (array with subset deleted=w477:T13)  [unwired: 1 in, 1 out]
          n196 = in-place-cluster #4("WatchList"=w477) -> (w474:T7)
        }
        n197 = Enqueue Element(queue=w470, element="update poll list") -> (queue out=w469:refnum<queue>)  [unwired: 2 in, 2 out]
        n198 = Enqueue Element(queue=w469, element="update UI") -> ()  [unwired: 2 in, 3 out]
      }
      frame "validate watch" {
        n199 = property class="MB PLC"(reference=w488) -> (reference out=w480:refnum<class "MB PLC Client.lvclass">, "Properties:PLC Config"=w487:T9)  [unwired: 1 in, 1 out]
        n200 = Unbundle By Name(w487) -> ("Reference Format"=w486:u16)
        n201 = local read "Starting Reference"() -> (w485:u32)
        n202 = local read "Data Type"() -> (w482:T4)
        n203 = call "Ref to Address.vi"("Reference"=w485, "Reference Format"=w486) -> ("Reference Type"=w483:T14)  [unwired: 8 in, 1 out]
        n204 = Format Into String(w483) -> (resulting string=→"Register Type":string)  [unwired: 3 in, 1 out]
        n205 = case shown="\"Coil\", Default" w483 {
          tunnel: w482 -> [_ w491]
          tunnel: [MB_Data_Types_Enum."Bool" ("Data Type") w491] -> w481
          frame "Coil", Default {
          }
          frame "Input Register", "Holding Register" {
          }
        }
        n206 = local write "Data Type"(w481) -> ()
      }
      frame "update poll list" {
        n207 = Unbundle By Name(w494) -> ("WatchList"=w500:T13)
        n208 = for {
          tunnel: w500 -> [w504] mode=indexing
          tunnel: [w501] -> w499 mode=indexing
          n209 = Unbundle By Name(w504) -> ("Reference"=w503:u32, "Data Type"=w502:T6)
          n210 = Bundle("Reference"=w503, "Data Type"=w502) -> (w501:cluster{"Reference":u32, "Data Type":T6})  [unwired: 1 in]
        }
        n211 = call "Generate Poll List.vi"("MaxPollGap"="MaxPollGap", "IO List"=w499) -> ("Poll List"=w495:T3[])  [unwired: 9 in]
        "Poll List" <- w495
        n212 = property class="MB PLC"(reference=w497, error in=w496, "Properties:Poll List"=w495) -> (reference out=w493:refnum<class "MB PLC Client.lvclass">, error out=w492:errorcluster)
      }
      frame "close" {
        n213 = call-dynamic "Close.vi"("error in (no error)"=w505, "PLC in"=w508) -> ("error out"=w506:errorcluster, "PLC out"=w507:refnum<class "MB PLC Client.lvclass">)  [unwired: 8 in]
        n214 = Bundle By Name(cluster=w511, "Open"=FALSE) -> (w509:T7)
      }
      frame "shutdown", Default {
        n215 = call-dynamic "Destruct.vi"("Destroy Data Block? (t)"=TRUE, "error in (no error)"=w517, "PLC in"=w518) -> ("error out"=w514:errorcluster)  [unwired: 8 in]
        n216 = Release Queue(queue=w513) -> ()  [unwired: 2 in, 3 out]
        n217 = Release Queue(queue=w512) -> ()  [unwired: 2 in, 3 out]
      }
    }
    n218 = case shown="Error" w70 {
      selector: w70 -> [w78 w87]
      tunnel: w69 -> [w80 w84]
      tunnel: w68 -> [w79 w81]
      tunnel: [w78 w86] -> w65
      tunnel: w64 -> [_ w85]
      tunnel: [w80 w82] -> w63
      tunnel: [w79 w81] -> w62
      frame No Error {
      }
      frame Error {
        n219 = Get Date/Time In Seconds() -> (seconds since 1Jan1904=w91:timestamp)
        n220 = Enqueue Element(queue=w85, element="close") -> ()  [unwired: 2 in, 3 out]
        n221 = Bundle By Name(cluster=w84, "Open"=FALSE) -> (w82:T7)
        n222 = call <vilib>:"Clear Errors.vi"("error in (no error)"=w87) -> ("error out"=w86:errorcluster)  [unwired: 5 in, 1 out]
        n223 = Format Date/Time String(time format string (%c)="%H:%M:%S%1u", seconds (now)=w91) -> (date/time string=→"Last Error Time":string)  [unwired: 1 in]
        "Last Error Status" <- w87
      }
    }
  }
